vi "Initialize Event Handler.vi"(1 "data queue":refnum<queue>) -> (0 "Event Refnum":refnum<event-registration>)   [LabVIEW 2018]
uses:
  Classes/Message/Message.lvclass
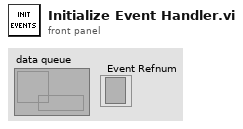
[diagram p1: front panel]
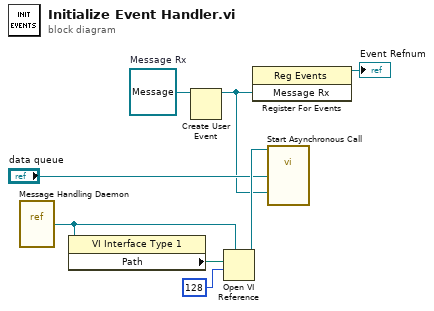
[diagram p0: block diagram]
diagram:
  w8 = refnum<class "Message.lvclass"> refnum  # Message Rx
  n1 = vi-ref "Message Handling Daemon.vi"() -> (w5:refnum<vi>)
  n2 = property class="VI Interface Type 1"(reference=w5) -> ("Path"=w7:path)  [unwired: 1 in, 2 out]
  n3 = Create User Event(user event datatype=w8) -> (user event=w2:refnum<user-event>)  [unwired: 1 in, 1 out]
  n4 = Open VI Reference(type specifier VI Refnum (for type only)=w5, vi path=w7, options=128) -> (vi reference=w4:refnum<vi>)  [unwired: 3 in, 1 out]
  n5 = register-events(w2) -> (reference out=→"Event Refnum":refnum<event-registration>)  [unwired: 2 in, 1 out]
  n6 = call-by-ref "Start Asynchronous Call"(reference=w4, "message event"=w2, "message queue"="data queue") -> ()  [unwired: 2 in, 2 out]
